vi "写入参数.vi"(8 "Error in":errorcluster caption="Error in (no error)", 9 "values":u16[](array[numeric]), 10 "starting address":u16, 11 "Slave ID":u8=10) -> (0 "error out":errorcluster)   [LabVIEW 2016, in "质控单元.lvlib"]
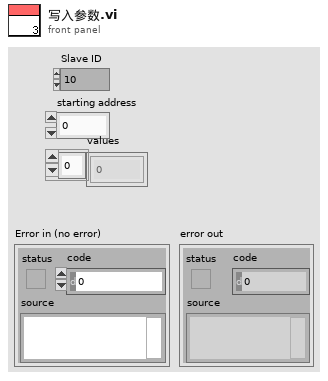
[diagram p1: front panel]
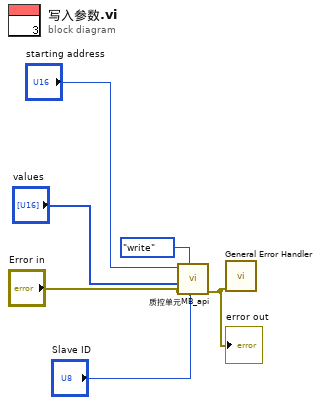
[diagram p0: block diagram]
diagram:
  n1 = call "质控单元MB_api.vi"("Slave ID"="Slave ID", "STEP"=enum16{"open", "read", "write", "close"}."write", "Error in"="Error in", "values"="values", "starting address"="starting address") -> ("error out"=w5:errorcluster)  [unwired: 3 in, 3 out]
  "error out" <- w5
  n2 = call <vilib>:"General Error Handler.vi"("error in (no error)"=w5) -> ()  [unwired: 10 in, 5 out]
